vi "LeggiDB.vi"(0 "Table":refnum<vi>, 1 "Inizio":timestamp format="%<%Y-%m-%d %H:%M>T", 2 "fine":timestamp format="%<%Y-%m-%d %H:%M>T") -> ()   [LabVIEW 2018]
uses:
  D:/LIBRERIE_LV/SQLite/subvi/TypeDef/Tipo_sqlite_open.ctl
  D:/LIBRERIE_LV/SQLite/sqlite3.lvlib
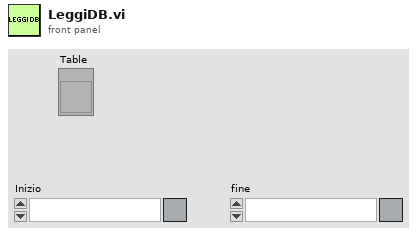
[diagram p1: front panel]
types:
  T1 = typedef "sqlite3.lvlib/Tipo_sqlite_open.ctl" = enum16{"file", "in memory"}
  T2 = cluster{"Query result[0]":string, "Query result[1]":string, "Query result[2]":string, "Query result[3]":string, "Query result[4]":string}
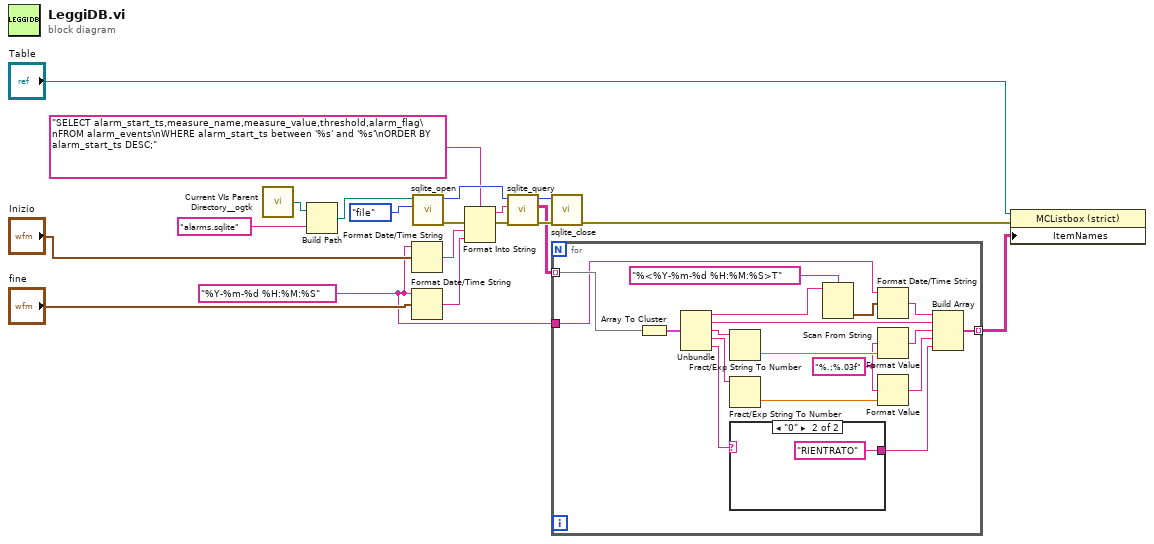
[diagram p0: block diagram]
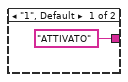
[diagram p2: hidden frame]
diagram:
  w5 = "%Y-%m-%d %H:%M:%S"
  n1 = call <userlib>:"Current VIs Parent Directory__ogtk.vi"() -> ("Parent Directory (+ Relative)"=w18:path)  [unwired: 5 in]
  n2 = Build Path(base path=w18, name or relative path="alarms.sqlite") -> (appended path=w17:path)
  n3 = Format Date/Time String(time format string (%c)=w5, seconds (now)="Inizio") -> (date/time string=w4:string)  [unwired: 1 in]
  n4 = Format Date/Time String(time format string (%c)=w5, seconds (now)="fine") -> (date/time string=w3:string)  [unwired: 1 in]
  n5 = call "sqlite_open.vi"("mode"=Tipo_sqlite_open."file", "Path"=w17) -> ("error out"=w2:errorcluster, "ppDb"=w20:u32)  [unwired: 8 in]
  n6 = Format Into String(format string="SELECT alarm_start_ts,measure_name,measure_value,threshold,alarm_flag\nFROM alarm_events\nWHERE alarm_start_ts between '%s' and '%s'\nORDER BY alarm_start_ts DESC;", error in=w2, w4, w3) -> (resulting string=w8:string, error out=w1:errorcluster)  [unwired: 1 in]
  n7 = call "sqlite_query.vi"("error in (no error)"=w1, "Query"=w8, "db in"=w20) -> ("error out"=w14:errorcluster, "Query result"=w13:string[][], "db out"=w19:u32)  [unwired: 6 in]
  n8 = call "sqlite_close.vi"("error in (no error)"=w14, "db in"=w19) -> ("error out"=w10:errorcluster)  [unwired: 9 in]
  n9 = for {
    tunnel: w13 -> [w38] mode=indexing
    tunnel: [w32] -> w12 mode=indexing
    tunnel: w5 -> [w21]
    w26 = "%.;%.03f" ("format string")
    n10 = Array To Cluster(array=w38) -> (cluster=w37:T2)
    n11 = Unbundle(w37) -> ("Query result[0]"=w36:string, "Query result[1]"=w31:string, "Query result[2]"=w30:string, "Query result[3]"=w25:string, "Query result[4]"=w23:string)
    n12 = Fract/Exp String To Number(string=w30) -> (number=w29:dbl)  [unwired: 3 in, 1 out]
    n13 = Fract/Exp String To Number(string=w25) -> (number=w27:dbl)  [unwired: 3 in, 1 out]
    n14 = case shown="\"0\"" w23 {
      tunnel: ["ATTIVATO" "RIENTRATO"] -> w22
      frame "1", Default {
      }
      frame "0" {
      }
    }
    n15 = Scan From String(format string="%<%Y-%m-%d %H:%M:%S>T", input string=w36) -> (output 1=w35:timestamp)  [unwired: 3 in, 3 out]
    n16 = Format Date/Time String(time format string (%c)=w21, seconds (now)=w35) -> (date/time string=w33:string)  [unwired: 1 in]
    n17 = Format Value(format string=w26, value (0)=w29) -> (output string=w28:string)  [unwired: 1 in]
    n18 = Format Value(format string=w26, value (0)=w27) -> (output string=w24:string)  [unwired: 1 in]
    n19 = Build Array(w33, w31, w28, w24, w22) -> (w32:string[])
  }
  n20 = property class="MCListbox (strict)"(reference="Table", error in=w10, "ItemNames"=w12) -> ()  [unwired: 2 out]
